vi "SyncPump_PID.vi"(0 "Control Enable":bool, 1 "Fault Input":bool, 2 "Rail Press Setpoint":sgl format="%.2f", 3 "Rail Pressure":sgl format="%.2f", 5 "PID Enable":bool, 9 "PID Settings":T4={"PID_Kp"=0.0, "PID_Ti"=0.01, "PID_Td"=0.0, "PID_FF"=0.0, "Non-PID_FF"=0.0, "PID_Min"=-100.0, "PID_Max"=100.0} {"PID_Max" format="%.2f"; "PID_Min" format="%.2f"; "PID_Td" format="%.3f"; "PID_Ti" format="%.3f"}, 11 "Output Management Controls":T2, 12 "dt (s)":sgl=-1.0 format="%.3f") -> (8 "Output":T1, 14 "PID_Action_Output":T3)   [LabVIEW 2015, in "ECS-RT.lvlib"]
uses:
  ECS-RT.lvlib
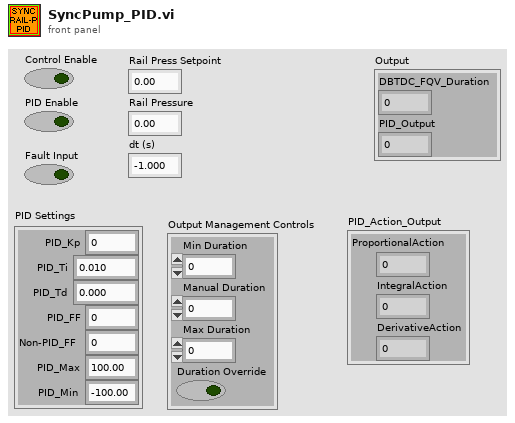
[diagram p1: front panel]
types:
  T1 = cluster{"DBTDC_FQV_Duration":sgl, "PID_Output":sgl}
  T2 = cluster{"Min Duration":sgl, "Manual Duration":sgl, "Max Duration":sgl, "Duration Override":bool}
  T3 = cluster{"ProportionalAction":sgl, "IntegralAction":sgl, "DerivativeAction":sgl}
  T4 = cluster{"PID_Kp":sgl, "PID_Ti":sgl, "PID_Td":sgl, "PID_FF":sgl, "Non-PID_FF":sgl, "PID_Min":sgl, "PID_Max":sgl}
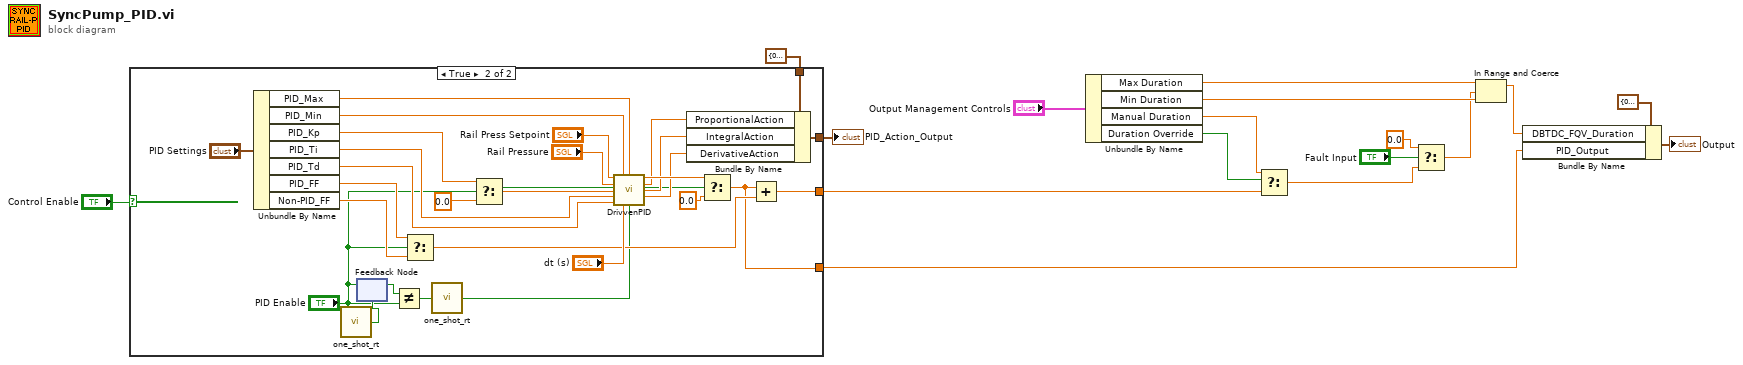
[diagram p0: block diagram]
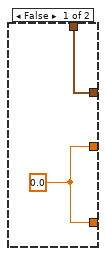
[diagram p2: hidden frame]
diagram:
  n1 = case shown="True" "Control Enable" {
    tunnel: [w19 w39] -> w16
    tunnel: [w19 w36] -> w17
    tunnel: T3 {"ProportionalAction"=0.0, "IntegralAction"=0.0, "DerivativeAction"=0.0} -> [w18 w25]
    tunnel: [w18 w24] -> w13
    frame False {
      w19 = sgl 0.0 ("f")
    }
    frame True {
      n2 = Unbundle By Name("PID Settings") -> ("PID_Max"=w32:sgl, "PID_Min"=w31:sgl, "PID_Kp"=w33:sgl, "PID_Ti"=w30:sgl, "PID_Td"=w29:sgl, "PID_FF"=w28:sgl, "Non-PID_FF"=w27:sgl)
      n3 = call <vilib>:"one_shot_rt.vi"("I"="PID Enable") -> ("O"=w21:bool)
      n4 = feedback #1(w21) -> (w38:bool)
      n5 = feedback-in #1("PID Enable") -> ()
      n6 = Not Equal?(x=w38, y="PID Enable") -> (x != y?=w37:bool)
      n7 = Select(t=w28, s="PID Enable", f=w27) -> (s? t:f=w42:sgl)
      n8 = call <vilib>:"one_shot_rt.vi"("I"=w37) -> ("O"=w35:bool)
      n9 = Select(t=w33, s="PID Enable", f=sgl 0.0 ("t")) -> (s? t:f=w46:sgl)
      n10 = call <vilib>:"DrivvenPID.vi"("Setpoint"="Rail Press Setpoint", "OutputLow"=w31, "OutputHigh"=w32, "ProcessVariable"="Rail Pressure", "ProportionalGain (Kc)"=w46, "IntegralTime (Ti, min)"=w30, "DerivativeTime (Td, min)"=w29, "dt (s)"="dt (s)", "Reinitialize? (F)"=w35) -> ("Output"=w41:sgl, "ProportionalAction"=w26:sgl, "IntegralAction"=w23:sgl, "DerivativeAction"=w22:sgl)  [unwired: 1 in, 2 out]
      n11 = Bundle By Name(cluster=w25, "ProportionalAction"=w26, "IntegralAction"=w23, "DerivativeAction"=w22) -> (w24:T3)
      n12 = Select(t=w41, s="PID Enable", f=sgl 0.0) -> (s? t:f=w39:sgl)
      n13 = Add(x=w39, y=w42) -> (x+y=w36:sgl)
    }
  }
  "PID_Action_Output" <- w13
  n14 = Unbundle By Name("Output Management Controls") -> ("Max Duration"=w11:sgl, "Min Duration"=w10:sgl, "Manual Duration"=w9:sgl, "Duration Override"=w15:bool)
  n15 = Select(t=w9, s=w15, f=w17) -> (s? t:f=w3:sgl)
  n16 = Select(t=sgl 0.0, s="Fault Input", f=w3) -> (s? t:f=w1:sgl)
  n17 = In Range and Coerce(upper limit=w11, x=w1, lower limit=w10) -> (coerced(x)=w8:sgl)  [unwired: 1 out]
  n18 = Bundle By Name(cluster=T1 {"DBTDC_FQV_Duration"=0.0, "PID_Output"=0.0} ("Output"), "DBTDC_FQV_Duration"=w8, "PID_Output"=w16) -> (→"Output":T1)
